vi "torque_creation.vi"(9 "duration":dbl, 10 "start":dbl, 11 "peak":dbl) -> (3 "torques":dbl[](array[numeric]))   [LabVIEW 2018]
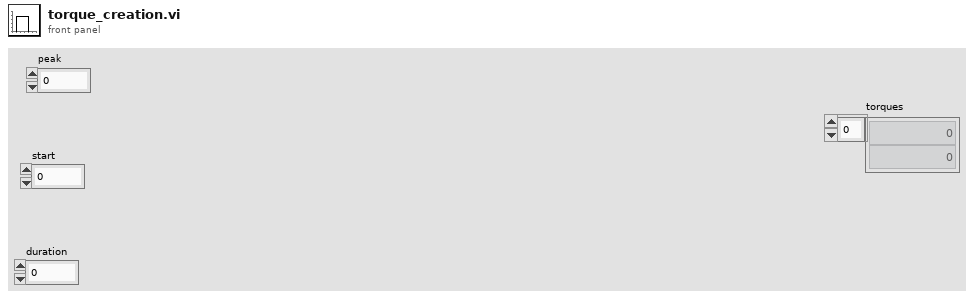
[diagram p1: front panel]
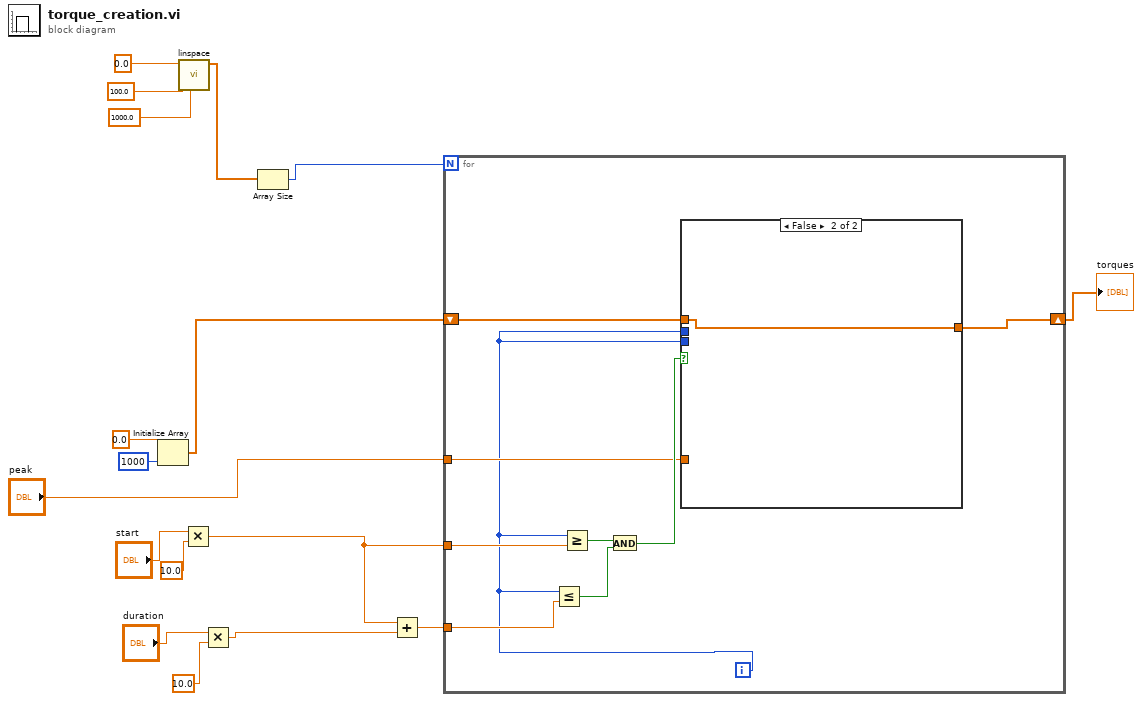
[diagram p0: block diagram]
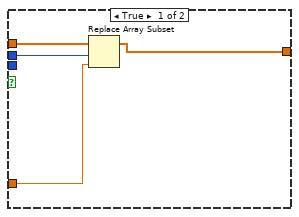
[diagram p2: hidden frame]
diagram:
  n1 = Initialize Array(0.0 ("element"), 1000 ("dimension size")) -> (w9:dbl[])
  n2 = call "linspace.vi"("NumElements"=1000.0, "End"=100.0, "Start"=0.0) -> ("Array"=w8:dbl[])  [unwired: 8 in]
  n3 = Multiply(x="start", y=10.0) -> (x*y=w4:dbl)
  n4 = Multiply(x="duration", y=10.0) -> (x*y=w1:dbl)
  n5 = Array Size(array=w8) -> (size(s)=w12:i32)
  n6 = Add(x=w4, y=w1) -> (x+y=w11:dbl)
  n7 = for {
    N: w12 -> [_]
    tunnel: w4 -> [w26]
    tunnel: w11 -> [w25]
    tunnel: "peak" -> [w21]
    shift-right: [w20] -> w7
    shift-left: w9 -> [w19]
    i -> [w18]
    n8 = Less Or Equal?(x=w18, y=w25) -> (x <= y?=w24:bool)
    n9 = Greater Or Equal?(x=w18, y=w26) -> (x >= y?=w23:bool)
    n10 = And(x=w23, y=w24) -> (x .and. y?=w22:bool)
    n11 = case shown="False" w22 {
      tunnel: w18 -> [w30 _]
      tunnel: w21 -> [w29 _]
      tunnel: w19 -> [w28 w31]
      tunnel: [w27 w31] -> w20
      tunnel: w18 -> [_ _]
      frame True {
        n12 = Replace Array Subset "Replace Array Subset"(array=w28, new element=w29, index=w30) -> (w27:dbl[])
      }
      frame False {
      }
    }
  }
  "torques" <- w7
